vi "Ferramenta de identificação.vi"() -> ()   [LabVIEW 2015]
panel:
  in  "Ordem do sistema":i32=4
  in  "Valor inicial das bombas":dbl=5.3
  out "subarray 3":dbl[][](array[numeric])
  in  "Identificar":bool
  in  "File Path Control":path
  out "Output 2":dbl[][](graph)
  out "Estimated MIMO State-space Model":picture
  out "Output 1":dbl[][](graph)
  # "Identificação da Planta"
  # "Escolha o arquivo excel gerado após a aquisição dos dados de excitação e resposta"
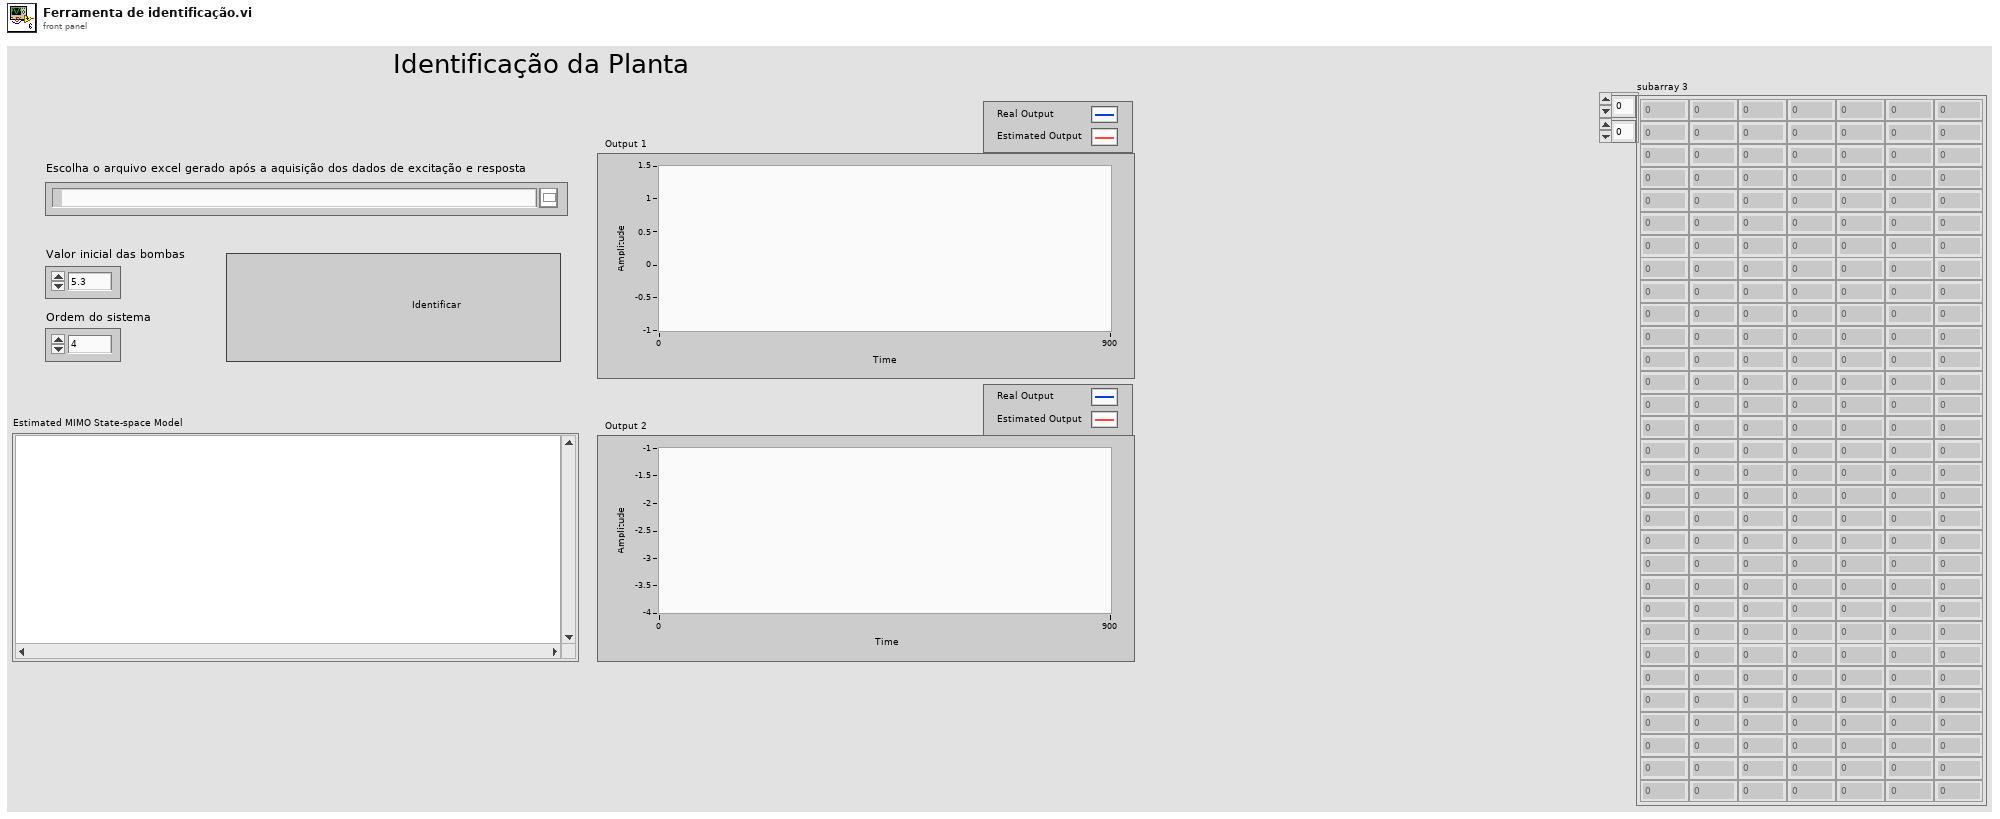
[diagram p1: front panel]
types:
  T1 = enum16{"Initialization", "Wait for event", "Read data", "Identification", "Close"}
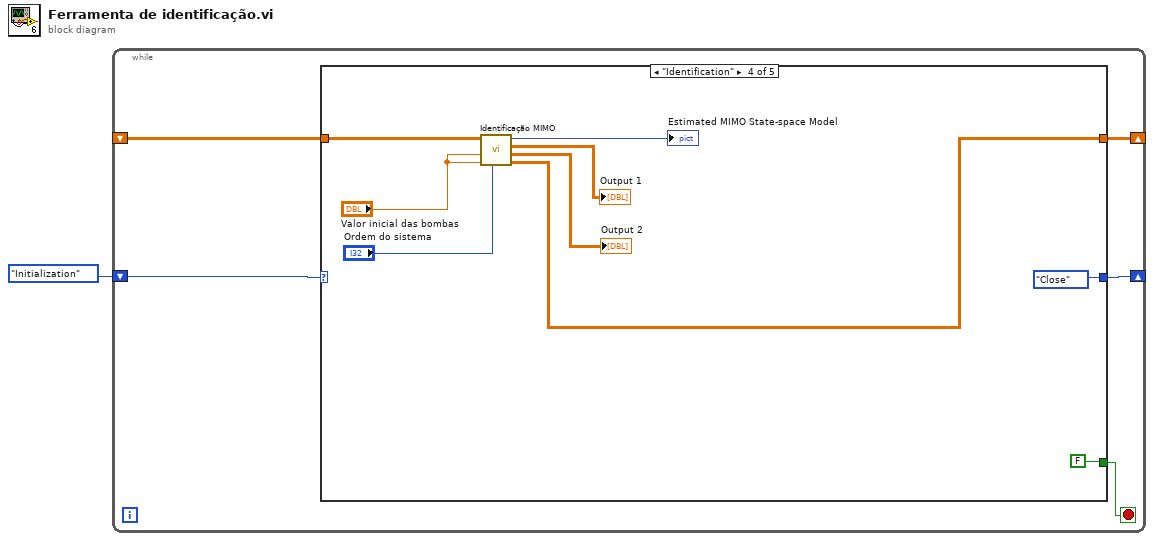
[diagram p0: block diagram]
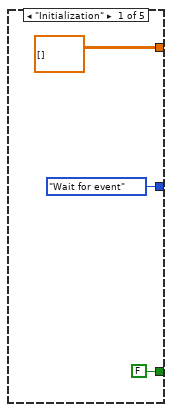
[diagram p2: hidden frame]
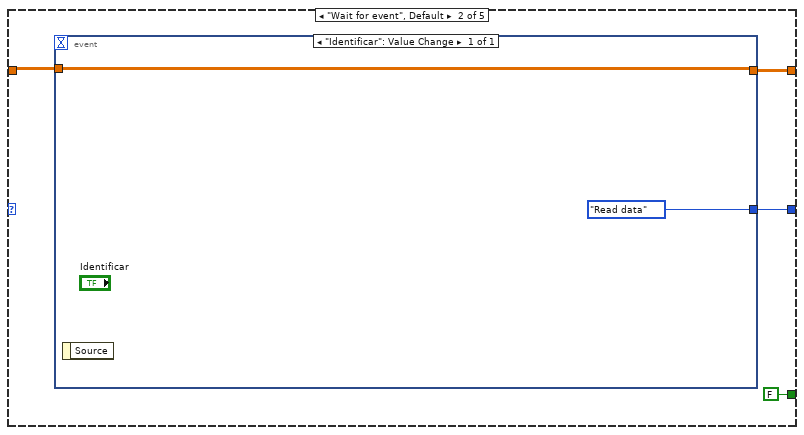
[diagram p3: hidden frame]
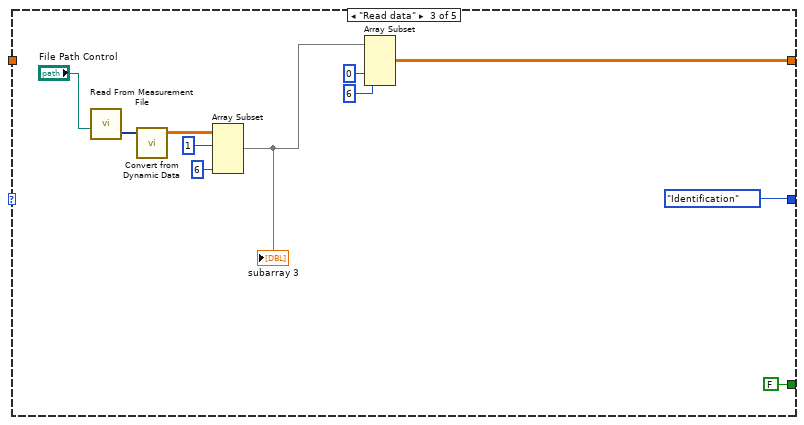
[diagram p4: hidden frame]
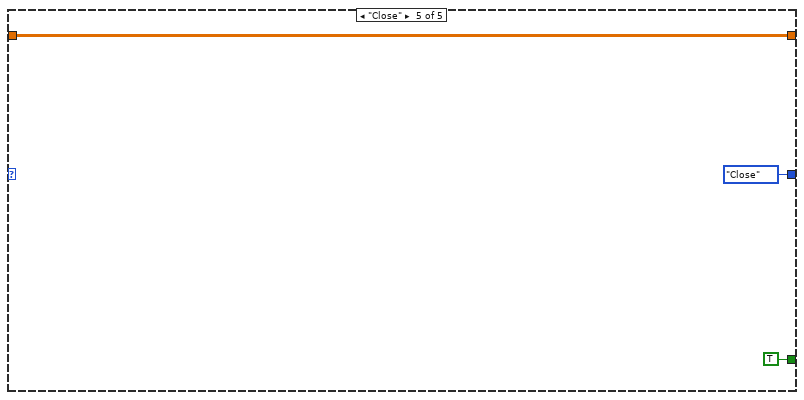
[diagram p5: hidden frame]
diagram:
  n1 = while {
    shift-right: [w5] -> _
    shift-left: T1."Initialization" -> [w6]
    shift-right: [w3] -> _
    shift-left: _ -> [w2]
    stop <- w4 stop-if-true
    n2 = case shown="\"Identification\"" w6 {
      tunnel: [T1."Wait for event" w13 T1."Identification" T1."Close" T1."Close"] -> w5
      tunnel: [FALSE FALSE FALSE FALSE TRUE] -> w4
      tunnel: [dbl[][] [] w11 w16 w27 w36] -> w3
      tunnel: w2 -> [_ w10 _ w33 w36]
      frame "Initialization" {
      }
      frame "Wait for event", Default {
        n3 = event shown="[0] \"Identificar\": Value Change" {
          selector: _ -> [_]
          dyn-events: _ -> [_]
          timeout: _ -> [_]
          tunnel: [T1."Read data"] -> w13
          tunnel: [w14] -> w11
          tunnel: w10 -> [w14]
          event "Identificar": Value Change {
            n4 = event-data() -> ()  [unwired: 1 in, 1 out]
          }
        }
      }
      frame "Read data" {
        n5 = call "Read From Measurement File"("Filename"="File Path Control") -> ("Signals"=w23:dynamicdata)  [unwired: 5 in, 5 out]
        n6 = call "Convert from Dynamic Data"("Dynamic Data Type"=w23) -> ("Array"=w22:dbl[][])  [unwired: 3 in]
        n7 = Array Subset(array=w22, index (row)=1 ("index"), length (col)=6 ("length")) -> (w17:dbl[][])  [unwired: 2 in]
        "subarray 3" <- w17
        n8 = Array Subset(array=w17, index (col)=0 ("index"), length (col)=6 ("length")) -> (w16:dbl[][])  [unwired: 2 in]
      }
      frame "Identification" {
        n9 = call "Identificação MIMO.vi"("System Order"="Ordem do sistema", "Init Pump 2 voltage"="Valor inicial das bombas", "Init Pump 1 voltage"="Valor inicial das bombas", "Stimulus and Response Signal"=w33) -> ("Acquired and identification signals"=w27:dbl[][], "output 2"=→"Output 2":dbl[][], "output 1"=→"Output 1":dbl[][], "Estimated MIMO State-space Model"=→"Estimated MIMO State-space Model":picture)  [unwired: 3 in, 1 out]
      }
      frame "Close" {
      }
    }
  }
